vi "SunyeeTestMain - Copy.vi"() -> ()   [LabVIEW 2018]
uses:
  <vilib>/Utility/error.llb/DialogType.ctl
  <vilib>/DAQmx/write.llb/DAQmx Write (Analog 1D Wfm NChan NSamp).vi
  <vilib>/DAQmx/create/channels.llb/DAQmx Create Channel (AO-Voltage-Basic).vi
  <vilib>/DAQmx/configure/timing.llb/DAQmx Timing (Sample Clock).vi
  <vilib>/Waveform/WDTOps.llb/WDT Append Waveforms DBL.vi
  <vilib>/DAQmx/miscellaneous.llb/DAQmx Fill In Error Info.vi
  <resource>/objmgr/daqmx.rc
panel:
  out "Waveform Graph 2":waveform(dbl)(graph)
  out "AO Actual Sample Rate":dbl=1000.0 format="%0.2f"
  in  "error in":errorcluster
  out "Waveform Graph2":waveform(dbl)(graph)
  out "Waveform Graph 1":waveform(dbl)(graph)
  out "Waveform Graph":waveform(dbl)[](graph)
  in  "Stop":bool
  in  "Physical Channel(s)":tag="PXI1Slot4_2/ao0:7"
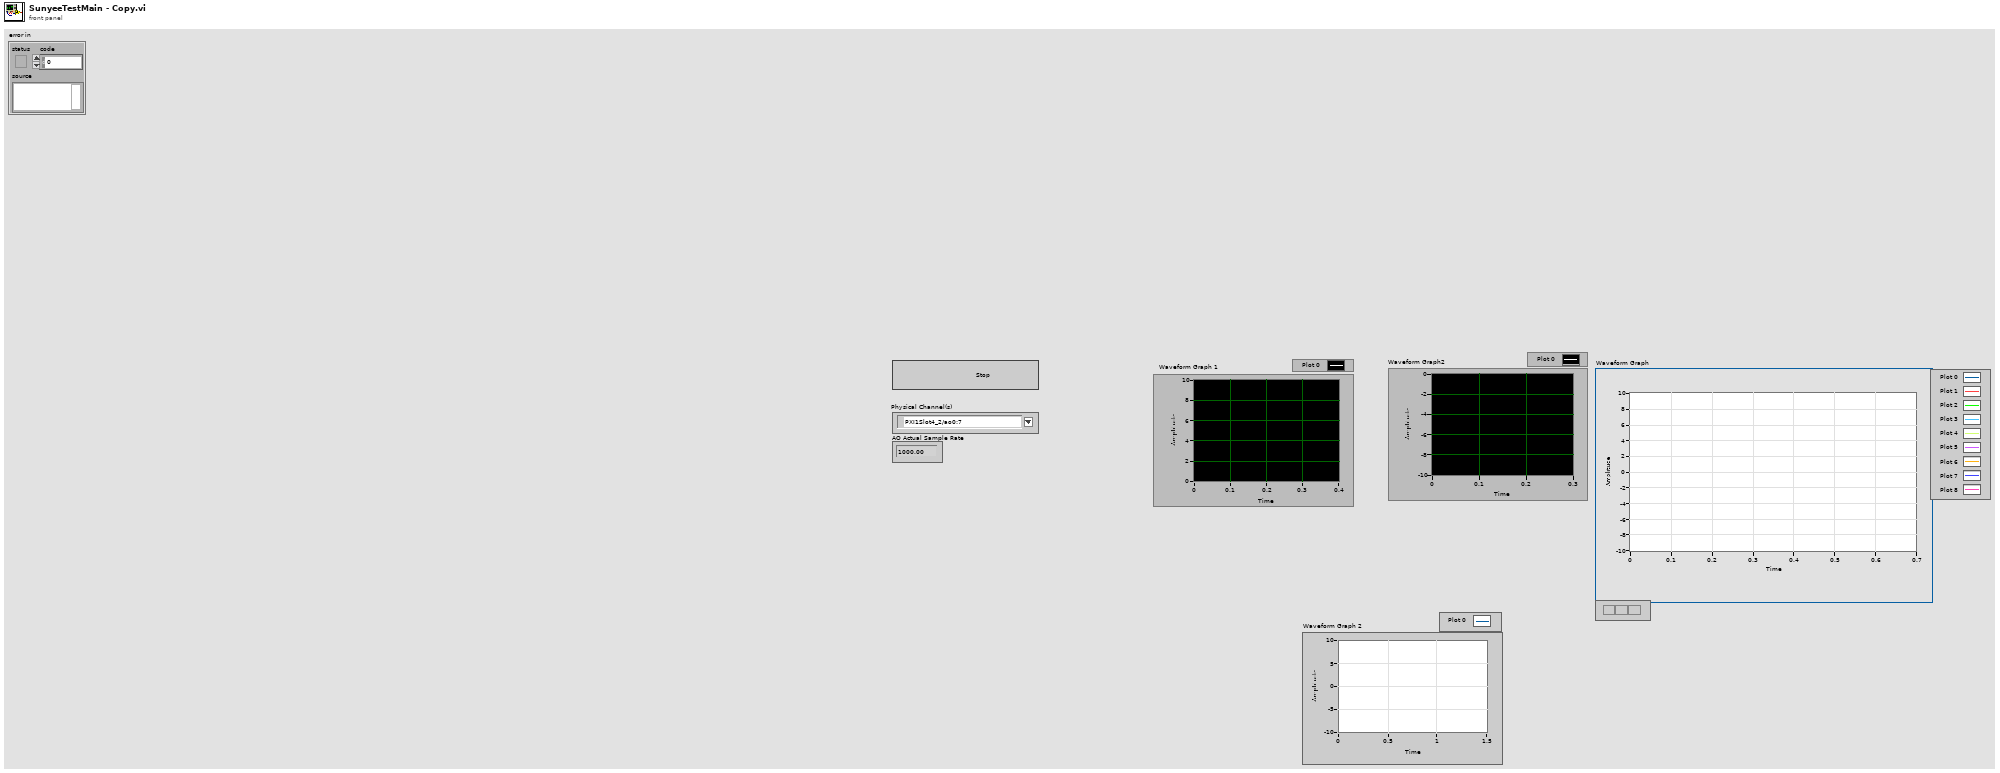
[diagram p1: front panel]
types:
  T1 = typedef "DialogType.ctl" = u16
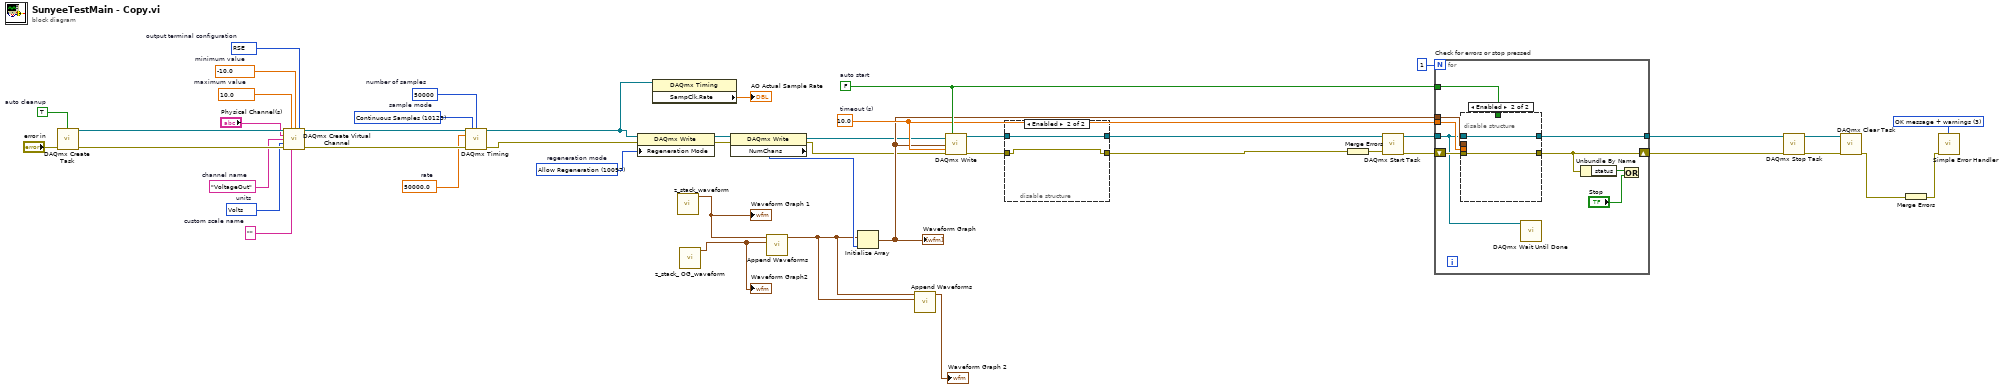
[diagram p0: block diagram]
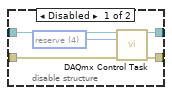
[diagram p2: hidden frame]
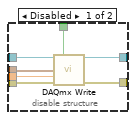
[diagram p3: hidden frame]
diagram:
  w24 = T1 3 items=["no dialog", "OK message", "continue or stop message", "OK message + warnings", "continue/stop + warnings"] ("type of dialog (OK msg:1)")
  w25 = 10097 items=["Allow Regeneration"=10097, "Do Not Allow Regeneration"=10158]  # regeneration mode
  w26 = 10123 items=["Finite Samples"=10178, "Continuous Samples"=10123, "Hardware Timed Single Point"=12522]  # sample mode
  w15 = 50000  # number of samples
  w27 = 50000.0  # rate
  w30 = 10083 items=["Default"=-1, "RSE"=10083, "Differential"=10106, "Pseudodifferential"=12529]  # output terminal configuration
  w31 = 10348 items=["Volts"=10348, "From Custom Scale"=10065]  # units
  w32 = "VoltageOut"  # channel name
  w34 = ""  # custom scale name
  w35 = -10.0  # minimum value
  w36 = 10.0  # maximum value
  w38 = TRUE  # auto cleanup
  w45 = 10.0  # timeout (s)
  w46 = FALSE  # auto start
  n1 = call <vilib>:"DAQmx Create Task.vi"("auto cleanup"=w38, "error in"="error in") -> ("task out"=w37:refnum<k21>, "error out"=w39:errorcluster)  [unwired: 12 in]
  n2 = call-poly <vilib>:"DAQmx Create Virtual Channel.vi"("task in"=w37, "maximum value"=w36, "minimum value"=w35, "output terminal configuration"=w30, "physical channels"="Physical Channel(s)", "name to assign"=w32, "units"=w31, "error in"=w39, "custom scale name"=w34) -> ("task out"=w28:refnum<k21>, "error out"=w33:errorcluster)  [unwired: 5 in]
  n3 = call-poly <vilib>:"DAQmx Timing.vi"("task/channels in"=w28, "sample mode"=w26, "samples per channel"=w15, "rate"=w27, "error in"=w33) -> ("task out"=w8:refnum<k21>, "error out"=w29:errorcluster)  [unwired: 9 in]
  n4 = property class="DAQmx Write"(reference=w8, error in=w29, "Regeneration Mode"=w25) -> (reference out=w13:refnum<k21>, error out=w12:errorcluster)
  n5 = property class="DAQmx Timing"(reference=w8) -> ("SampClk.Rate"=→"AO Actual Sample Rate":dbl)  [unwired: 1 in, 2 out]
  n6 = call "z_stack_waveform.vi"() -> ("waveform out"=w20:waveform(dbl))  [unwired: 9 in, 2 out]
  "Waveform Graph 1" <- w20
  n7 = call "z_stack_ OG_waveform.vi"() -> ("waveform out"=w19:waveform(dbl))  [unwired: 15 in, 4 out]
  "Waveform Graph2" <- w19
  n8 = property class="DAQmx Write"(reference=w13, error in=w12) -> (reference out=w11:refnum<k21>, error out=w10:errorcluster, "NumChans"=w9:u32)
  n9 = call-poly <vilib>:"Append Waveforms.vi"("waveform B"=w19, "waveform A"=w20) -> ("waveform out"=w2:waveform(dbl))  [unwired: 8 in, 1 out]
  n10 = Initialize Array(w2, w9) -> (w18:waveform(dbl)[])
  "Waveform Graph" <- w18
  n11 = call-poly <vilib>:"Append Waveforms.vi"("waveform B"=w2, "waveform A"=w2) -> ("waveform out"=→"Waveform Graph 2":waveform(dbl))  [unwired: 8 in, 1 out]
  n12 = call-poly <vilib>:"DAQmx Write.vi"("task/channels in"=w11, "auto start"=w46, "data"=w18, "timeout"=w45, "error in"=w10) -> ("task out"=w44:refnum<k21>, "error out"=w42:errorcluster)  [unwired: 8 in, 1 out]
  n13 = disable-structure shown="Enabled" {
    disable-tunnel: w44 -> [w52 w54]
    disable-tunnel: [w51 w54] -> w43
    disable-tunnel: w42 -> [w50 w53]
    disable-tunnel: [w49 w53] -> w17
    frame Disabled {
      w48 = 4 items=["verify"=2, "reserve"=4, "commit"=3, "unreserve"=5, "abort"=6] ("action")
      n14 = call <vilib>:"DAQmx Control Task.vi"("task/channels in"=w52, "action"=w48, "error in"=w50) -> ("task out"=w51:refnum<k21>, "error out"=w49:errorcluster)  [unwired: 11 in]
    }
    frame Enabled {
    }
  }
  n15 = Merge Errors(w17) -> (w16:errorcluster)
  n16 = call <vilib>:"DAQmx Start Task.vi"("task/channels in"=w43, "error in"=w16) -> ("task out"=w47:refnum<k21>, "error out"=w41:errorcluster)  [unwired: 12 in]
  n17 = for "Check for errors or stop pressed" {
    N: 1 -> [_]
    tunnel: [w63] -> w21
    tunnel: w47 -> [w55]
    shift-right: [w60] -> w5
    shift-left: w41 -> [w62]
    tunnel: w46 -> [w59]
    tunnel: w18 -> [w58]
    tunnel: w45 -> [w57]
    n18 = disable-structure shown="Enabled" {
      disable-tunnel: [w70 w72] -> w63
      disable-tunnel: w62 -> [w69 w71]
      disable-tunnel: [w68 w71] -> w60
      disable-tunnel: w59 -> [w67 _]
      disable-tunnel: w58 -> [w66 _]
      disable-tunnel: w57 -> [w65 _]
      disable-tunnel: w55 -> [w64 w72]
      frame Disabled {
        n19 = call-poly <vilib>:"DAQmx Write.vi"("task/channels in"=w64, "auto start"=w67, "data"=w66, "timeout"=w65, "error in"=w69) -> ("task out"=w70:refnum<k21>, "error out"=w68:errorcluster)  [unwired: 8 in, 1 out]
      }
      frame Enabled {
      }
    }
    n20 = call <vilib>:"DAQmx Wait Until Done.vi"("task/channels in"=w55) -> ()  [unwired: 13 in, 2 out]
    n21 = Unbundle By Name(w60) -> ("status"=w61:bool)
    n22 = Or(x=w61, y="Stop") -> ()  [unwired: 1 out]
  }
  n23 = call <vilib>:"DAQmx Stop Task.vi"("task/channels in"=w21, "error in"=w5) -> ("task out"=w22:refnum<k21>, "error out"=w23:errorcluster)  [unwired: 12 in]
  n24 = call <vilib>:"DAQmx Clear Task.vi"("task in"=w22, "error in"=w23) -> ("error out"=w4:errorcluster)  [unwired: 13 in]
  n25 = Merge Errors(w4) -> (w3:errorcluster)
  n26 = call <vilib>:"Simple Error Handler.vi"("type of dialog (OK msg:1)"=w24, "error in (no error)"=w3) -> ()  [unwired: 3 in, 5 out]
